vi "parameters-get.vi"(0 "Parameters":refnum<vi>, 5 "Time":dbl, 11 "error in (no error)":errorcluster) -> (4 "Parameter out":refnum<vi>, 6 "Samples":T1, 8 "Lambda":T1, 10 "Stabilizing":T1, 15 "error out":errorcluster)   [LabVIEW 2016]
uses:
  <vilib>/Utility/miscctls.llb/LVRangeTypeDef.ctl
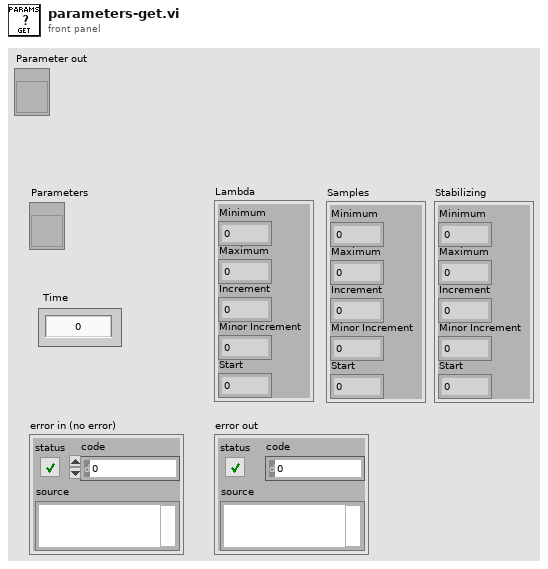
[diagram p1: front panel]
types:
  T1 = typedef "LVRangeTypeDef.ctl" = cluster{"Minimum":dbl, "Maximum":dbl, "Increment":dbl, "Minor Increment":dbl, "Start":dbl}
  T2 = typedef "Parameters.ctl" = cluster{"Lambda":T3, "Power":dbl, "Frequency":dbl, "Stabilizing":dbl, "Samples":dbl}
  T3 = typedef "Lambda.ctl" = cluster{"Init":dbl, "Final":dbl, "dx":dbl}
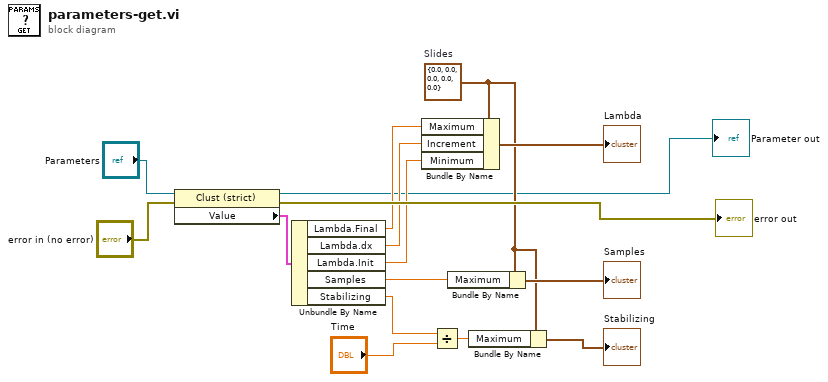
[diagram p0: block diagram]
diagram:
  w6 = T1 {"Minimum"=0.0, "Maximum"=0.0, "Increment"=0.0, "Minor Increment"=0.0, "Start"=0.0}  # Slides
  n1 = property class="Clust (strict)"(reference="Parameters", error in="error in (no error)") -> (reference out=→"Parameter out":refnum<vi>, error out=→"error out":errorcluster, "Value"=w12:T2)
  n2 = Unbundle By Name(w12) -> ("Lambda.Final"=w13:dbl, "Lambda.dx"=w10:dbl, "Lambda.Init"=w9:dbl, "Samples"=w7:dbl, "Stabilizing"=w4:dbl)
  n3 = Bundle By Name(cluster=w6, "Maximum"=w13, "Increment"=w10, "Minimum"=w9) -> (→"Lambda":T1)
  n4 = Divide(x=w4, y="Time") -> (x/y=w3:dbl)
  n5 = Bundle By Name(cluster=w6, "Maximum"=w7) -> (→"Samples":T1)
  n6 = Bundle By Name(cluster=w6, "Maximum"=w3) -> (→"Stabilizing":T1)
